vi "get temperature.vi"(8 "error in":errorcluster) -> (0 "error out":errorcluster, 2 "temperature [ºC]":dbl)   [LabVIEW 2013]
uses:
  <vilib>/myRIO/Instrument Drivers/Onboard IO/I2C/vis/Smart Open.vi
  <vilib>/myRIO/Instrument Drivers/Onboard IO/I2C/vis/Configure.vi
  <vilib>/myRIO/Instrument Drivers/Onboard IO/I2C/vis/Write.vi
  <vilib>/myRIO/Instrument Drivers/Onboard IO/I2C/vis/Read.vi
  <vilib>/myRIO/Instrument Drivers/Onboard IO/I2C/vis/Open.vi
  <vilib>/myRIO/Common/Instrument Driver Framework/myRIO v1.0/I2C/vis/myRIO v1.1 Open I2C.vi
  <vilib>/myRIO/Common/Instrument Driver Framework/Utilities/vis/Validate Channels.vi
  <vilib>/myRIO/Common/Instrument Driver Framework/myRIO v1.0/I2C/vis/myRIO v1.0 Reserve I2C.vi
  <vilib>/myRIO/Common/Instrument Driver Framework/myRIO v1.0/I2C/vis/myRIO v1.0 Build MUX Configuration I2C.vi
  <vilib>/myRIO/Common/Instrument Driver Framework/myRIO v1.0/Resource Manager/vis/myRIO v1.0 Reserve Channel List.vi
  <vilib>/myRIO/Common/Instrument Driver Framework/myRIO v1.0/Resource Manager/vis/myRIO v1.0 Create Configuration List.vi
  <vilib>/myRIO/Common/Instrument Driver Framework/myRIO v1.0/Resource Manager/vis/myRIO v1.0 Reserve Channel.vi
  <vilib>/myRIO/Common/Instrument Driver Framework/myRIO v1.0/Resource Manager/vis/myRIO v1.0 Unreserve Channel.vi
  <vilib>/myRIO/Common/Instrument Driver Framework/myRIO v1.0/Resource Manager/vis/myRIO v1.0 Build Mutex Name.vi
  <vilib>/myRIO/Common/Instrument Driver Framework/myRIO v1.0/myRIO v1.1 Open.vi
  <vilib>/Utility/VariantDataType/GetNumericInfo.vi
  <vilib>/Utility/error.llb/Error Cluster From Error Code.vi
  <vilib>/myRIO/Common/Instrument Driver Framework/Utilities/vis/IO Manager.vi
  <vilib>/myRIO/Common/Instrument Driver Framework/Utilities/vis/Configuration Manager.vi
  <vilib>/myRIO/Common/Instrument Driver Framework/myRIO v1.0/Resource Manager/vis/myRIO v1.0 Configure IO.vi
  <vilib>/myRIO/Common/Instrument Driver Framework/myRIO v1.0/myRIO v1.0 Close.vi
  <vilib>/myRIO/Common/Instrument Driver Framework/myRIO v1.0/I2C/vis/myRIO v1.0 Configure I2C.vi
  <vilib>/myRIO/Common/Instrument Driver Framework/myRIO v1.0/I2C/vis/myRIO v1.0 Write I2C.vi
  <vilib>/myRIO/Common/Instrument Driver Framework/myRIO v1.0/I2C/vis/myRIO v1.0 Read I2C.vi
panel:
  # "get temperature"
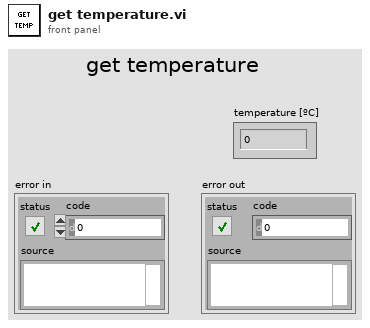
[diagram p1: front panel]
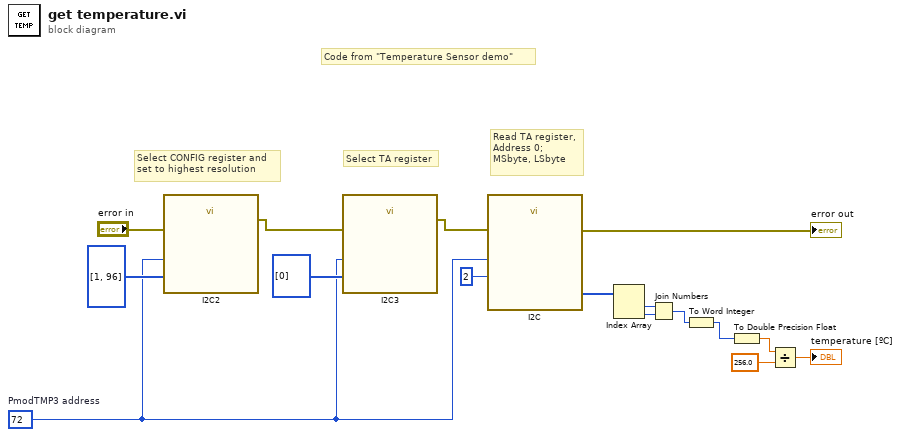
[diagram p0: block diagram]
diagram:
  w3 = u8 72  # PmodTMP3 address
  # "Select TA register"
  # "Select CONFIG register and\nset to highest resolution"
  # "Code from \"Temperature Sensor demo\""
  # "Read TA register,\nAddress 0;\nMSbyte, LSbyte"
  n1 = call "I2C2"("Slave Address (7-bit)"=w3, "Bytes to Write"=u8[] [1, 96], "error in (no error)"="error in") -> ("error out"=w2:errorcluster)  [unwired: 24 in]
  n2 = call "I2C3"("Slave Address (7-bit)"=w3, "Bytes to Write"=u8[] [0], "error in (no error)"=w2) -> ("error out"=w1:errorcluster)  [unwired: 24 in]
  n3 = call "I2C"("Slave Address (7-bit)"=w3, "Byte Count"=u32 2, "error in (no error)"=w1) -> ("Bytes Read"=w9:u8[], "error out"=→"error out":errorcluster)  [unwired: 23 in]
  n4 = Index Array "Index Array"(array=w9) -> (element #1=w14:u8, element #2=w13:u8)  [unwired: 2 in]
  n5 = Join Numbers(hi=w14, lo=w13) -> ((hi.lo)=w11:u16)
  n6 = To Word Integer(number=w11) -> (16bit integer=w10:i16)
  n7 = To Double Precision Float(number=w10) -> (double precision float=w16:dbl)
  n8 = Divide(x=w16, y=256.0) -> (x/y=→"temperature [ºC]":dbl)
